vi "SQL執行.vi"(0 "ConnectionString":string="Driver=SQL Server;Server=PPC-3XX0S;Database=scontroldb;uid=eliUser;pwd=eli$1234;", 7 "出資料":bool=TRUE, 9 "CommandText":string="SELECT * FROM  Gweight ;", 11 "error in (no error)":errorcluster) -> (4 "Data":string[][](array[string])=[["TH-32H400W", "2020/3/18 上午 11:53:10", "5750", "5550", "5854", "0"]], 15 "error out":errorcluster)   [LabVIEW 2014]
panel:
  in  "ADODB._Connection":refnum<k7>
  # "INSERT INTO tablename (id, hw, score) VALUES ('1234567', 2, 89)"
  # "SELECT CONVERT(char(19), getdate(), 120)"
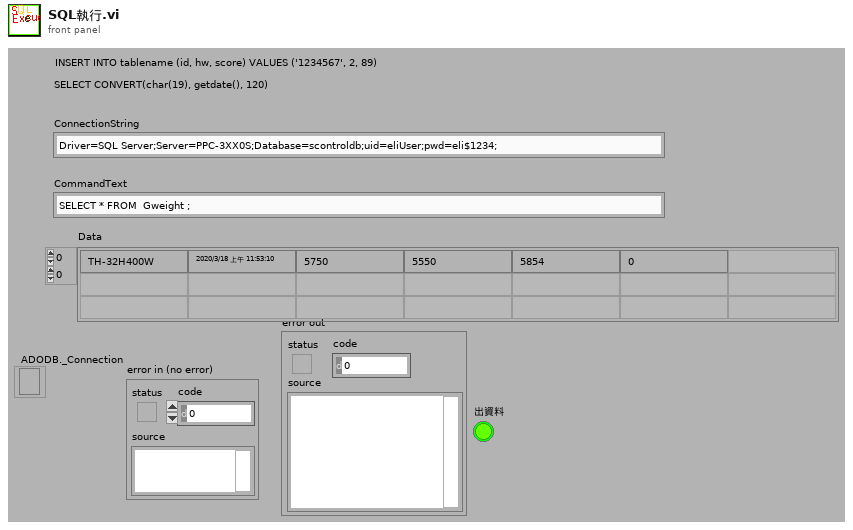
[diagram p1: front panel]
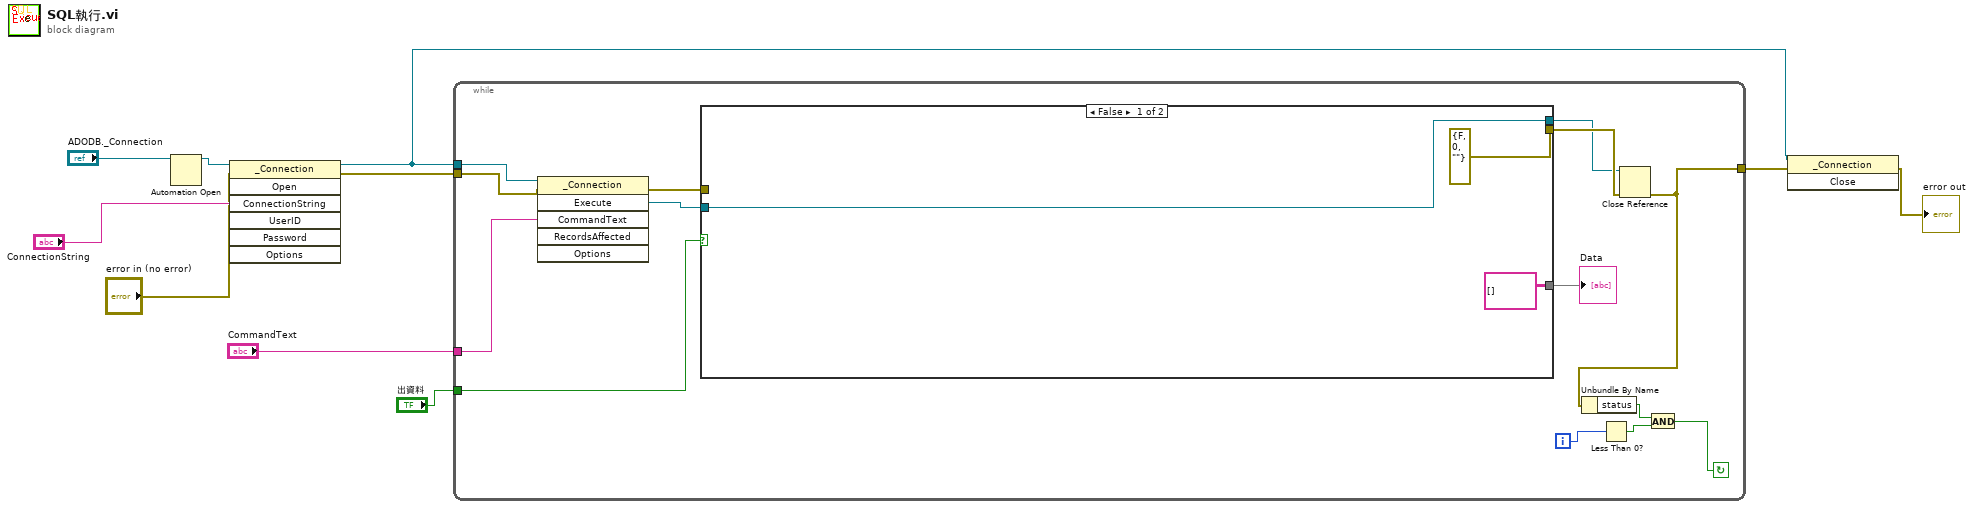
[diagram p0: block diagram]
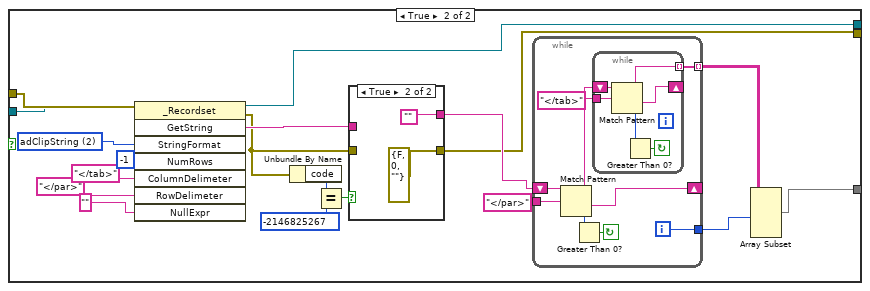
[diagram p2: hidden frame]
diagram:
  n1 = Automation Open(Automation Refnum="ADODB._Connection") -> (Automation Refnum=w6:refnum<k7>)  [unwired: 3 in, 1 out]
  n2 = invoke class="_Connection" method="Open"(reference=w6, error in="error in (no error)", "ConnectionString"="ConnectionString") -> (reference out=w1:refnum<k7>, error out=w7:errorcluster)  [unwired: 4 in, 5 out]
  n3 = while {
    tunnel: "CommandText" -> [w24]
    tunnel: w7 -> [w20]
    tunnel: w1 -> [w19]
    tunnel: "出資料" -> [w17]
    tunnel: [w11] -> w2
    i -> [w23]
    stop <- w21 continue-if-true
    n4 = invoke class="_Connection" method="Execute"(reference=w19, error in=w20, "CommandText"=w24) -> (error out=w14:errorcluster, "Execute"=w13:refnum<k7>)  [unwired: 3 in, 4 out]
    n5 = case shown="False" w17 {
      tunnel: [errorcluster {"status"=FALSE, "code"=0, "source"=""} ("error out") w32] -> w15
      tunnel: [string[][] [] w31] -> w16
      tunnel: w14 -> [_ w30]
      tunnel: w13 -> [w27 w29]
      tunnel: [w27 w28] -> w12
      frame False {
      }
      frame True {
        w46 = 2 items=["adClipString"=2] ("StringFormat")
        n6 = invoke class="_Recordset" method="GetString"(reference=w29, error in=w30, "StringFormat"=w46, "NumRows"=-1, "ColumnDelimeter"="</tab>", "RowDelimeter"="</par>", "NullExpr"="") -> (reference out=w28:refnum<k7>, error out=w38:errorcluster, "GetString"=w39:string)  [unwired: 1 in, 5 out]
        n7 = Unbundle By Name(w38) -> ("code"=w42:i32)
        n8 = Equal?(x=w42, y=-2146825267) -> (x = y?=w40:bool)
        n9 = case shown="True" w40 {
          tunnel: [w63 errorcluster {"status"=FALSE, "code"=0, "source"=""} ("error out")] -> w32
          tunnel: w38 -> [w63 _]
          tunnel: [w62 ""] -> w33
          tunnel: w39 -> [w62 _]
          frame False {
          }
          frame True {
          }
        }
        n10 = while {
          shift-left: w33 -> [w49]
          shift-right: [w48] -> _
          tunnel: "</par>" ("delimiter (Tab)") -> [w55]
          tunnel: [w53] -> w36
          tunnel: [w50] -> w34 mode=indexing
          i -> [w53]
          stop <- w54 continue-if-true
          n11 = Match Pattern(string=w49, regular expression=w55) -> (before substring=w47:string, after substring=w48:string, offset past match=w52:i32)  [unwired: 1 in, 1 out]
          n12 = Greater Than 0?(x=w52) -> (x > 0?=w54:bool)
          n13 = while {
            tunnel: "</tab>" ("delimiter (Tab)") -> [w56]
            tunnel: [w59] -> w50 mode=indexing
            shift-left: w47 -> [w61]
            shift-right: [w60] -> _
            stop <- w58 continue-if-true
            n14 = Match Pattern(string=w61, regular expression=w56) -> (before substring=w59:string, after substring=w60:string, offset past match=w57:i32)  [unwired: 1 in, 1 out]
            n15 = Greater Than 0?(x=w57) -> (x > 0?=w58:bool)
          }
        }
        n16 = Array Subset(array=w34, length (row)=w36) -> (w31:string[][])  [unwired: 3 in]
      }
    }
    "Data" <- w16
    n17 = Less Than 0?(x=w23) -> (x < 0?=w22:bool)
    n18 = Close Reference(reference=w12, error in (no error)=w15) -> (error out=w11:errorcluster)
    n19 = Unbundle By Name(w11) -> ("status"=w18:bool)
    n20 = And(x=w18, y=w22) -> (x .and. y?=w21:bool)
  }
  n21 = invoke class="_Connection" method="Close"(reference=w1, error in=w2) -> (error out=→"error out":errorcluster)  [unwired: 1 in, 2 out]
